vi "DMM Read Dual Display.vi"() -> ()   [LabVIEW 2018]
uses:
  <instrlib>/DMM4/DMM4.lvlib
panel:
  in  "measure":bool
  in  "Reset":bool=TRUE
  out "Measure 2nd Value":string
  in  "Manual Range":dbl=0.5 format="%#.9e"
  in  "Auto Range":bool
  in  "2nd Function":u8(ring)=2 items=["DC Voltage", "AC Voltage", "DC Current", "AC Current", "2-Wire Resistance", "Frequency", "Period", "None"]
  in  "1st Function":u8(ring) items=["DC Voltage", "AC Voltage", "DC+AC Voltage", "DC Current", "AC Current", "DC+AC Current", "2-Wire Resistance", "Frequency", "Period", "Continuity", "Diode", "Temperature", "Capacitance"]
  out "error out":errorcluster
  out "Measure 1st Value":string
  in  "Stop":bool
  out "Boolean":bool
  in  "Detector Rate":u16(ring)=2 items=["SLOW", "MID", "FAST"]
  in  "Manual Range":dbl=1000.0 format="%#.9e"
  in  "Auto Range":bool
  out "ID Return String":string
  in  "Configure RS232 Baud Rate":u32(ring)=115200 items=["9600"=9600, "19200"=19200, "38400"=38400, "57600"=57600, "115200"=115200]
  in  "VISA resource name":refnum<visa-resource-name>="COM15"
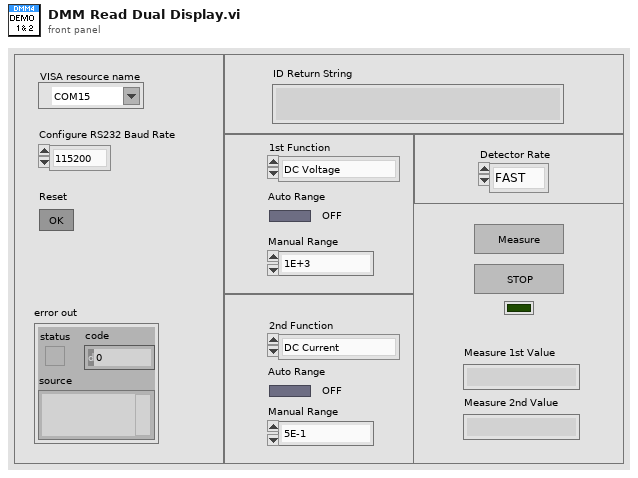
[diagram p1: front panel]
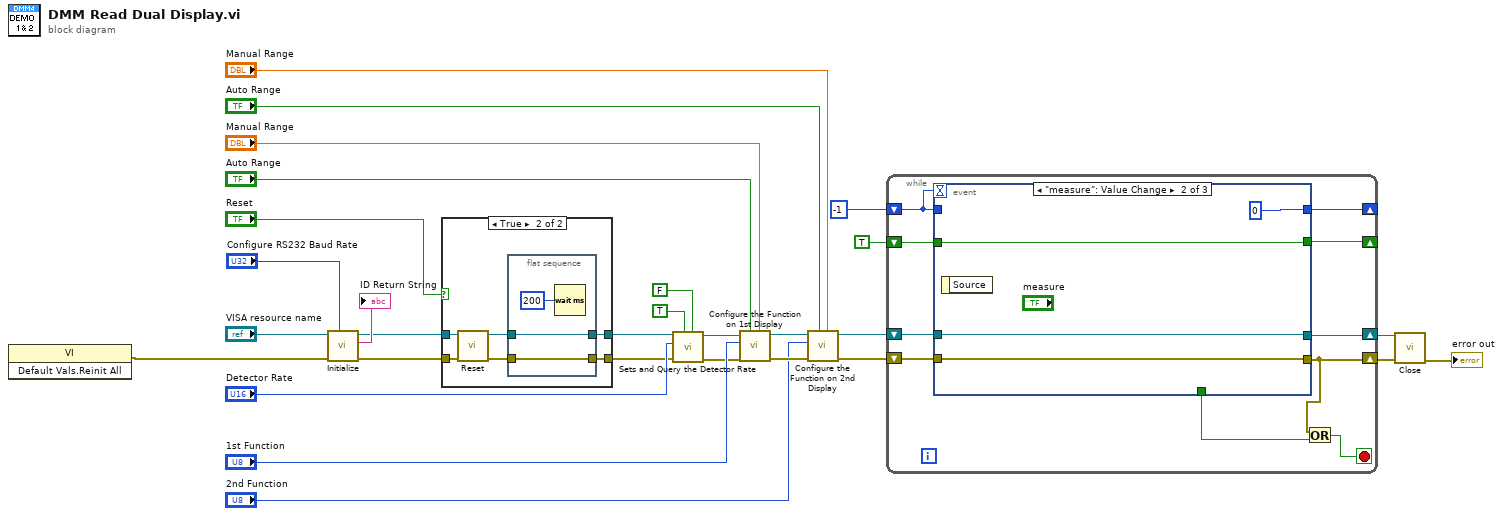
[diagram p0: block diagram]
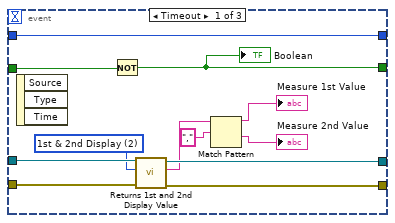
[diagram p3: hidden frame]
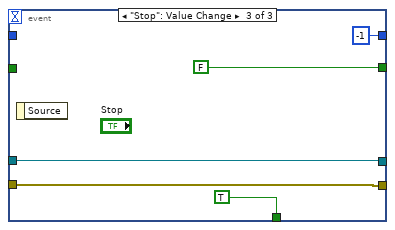
[diagram p4: hidden frame]
diagram:
  n1 = invoke class="VI" method="Default Vals.Reinit All"() -> (error out=w1:errorcluster)  [unwired: 3 in, 2 out]
  n2 = call <instrlib>:"Initialize.vi"("Configure RS232 Baud Rate"="Configure RS232 Baud Rate", "error in (no error)"=w1, "VISA resource name"="VISA resource name") -> ("error out"=w20:errorcluster, "ID Return String"=→"ID Return String":string, "VISA resource name out"=w21:refnum<visa-resource-name>)  [unwired: 5 in, 1 out]
  n3 = case shown="True" "Reset" {
    tunnel: w21 -> [w31 w37]
    tunnel: w20 -> [w30 w36]
    tunnel: [w31 w34] -> w4
    tunnel: [w30 w32] -> w3
    frame False {
    }
    frame True {
      n4 = call <instrlib>:"Reset.vi"("error in (no error)"=w36, "VISA resource name"=w37) -> ("error out"=w33:errorcluster, "VISA resource name out"=w35:refnum<visa-resource-name>)  [unwired: 8 in]
      n5 = flat-sequence {
        tunnel: w35 -> [w39]
        tunnel: [w39] -> w34
        tunnel: w33 -> [w38]
        tunnel: [w38] -> w32
        frame #0 {
          n6 = Wait (ms)(milliseconds to wait=u32 200) -> ()  [unwired: 1 out]
        }
      }
    }
  }
  n7 = call <instrlib>:"Sets and Query the Detector Rate.vi"("Enable to Query"=FALSE, "Enable to Sets"=TRUE, "error in"=w3, "Detector Rate"="Detector Rate", "VISA resource name"=w4) -> ("error out"=w9:errorcluster, "VISA resource name out"=w10:refnum<visa-resource-name>)  [unwired: 4 in, 1 out]
  n8 = call <instrlib>:"Configure the Function on 1st Display .vi"("Manual Range"="Manual Range", "Enable Auto Range"="Auto Range", "error in"=w9, "Function"="1st Function", "VISA resource name"=w10) -> ("error out"=w17:errorcluster, "VISA resource name out"=w18:refnum<visa-resource-name>)  [unwired: 5 in]
  n9 = call <instrlib>:"Configure the Function on 2nd Display.vi"("Manual Range"="Manual Range", "Enable Auto Range"="Auto Range", "error in"=w17, "Function"="2nd Function", "VISA resource name"=w18) -> ("error out"=w11:errorcluster, "VISA resource name out"=w12:refnum<visa-resource-name>)  [unwired: 5 in]
  n10 = while {
    shift-right: [w46] -> _
    shift-left: TRUE -> [w47]
    shift-right: [w44] -> _
    shift-left: -1 -> [w45]
    shift-right: [w48] -> w24
    shift-left: w12 -> [w50]
    shift-right: [w43] -> w23
    shift-left: w11 -> [w49]
    stop <- w41 stop-if-true
    n11 = event shown="[1] \"measure\": Value Change" {
      selector: _ -> [_ _ _]
      dyn-events: _ -> [_ _ _]
      timeout: w45 -> [_ _ _]
      tunnel: w50 -> [w62 w66 w71]
      tunnel: w49 -> [w61 w65 w69]
      tunnel: [w59 w66 w71] -> w48
      tunnel: [w58 w65 w69] -> w43
      tunnel: w47 -> [w57 w64 _]
      tunnel: [w56 w64 FALSE] -> w46
      tunnel: [_ _ TRUE] -> w42
      tunnel: w45 -> [w51 _ _]
      tunnel: [w51 0 -1] -> w44
      event Timeout {
        w60 = u16 2 items=["1st Display", "2nd Display", "1st & 2nd Display"] ("Sets to Display")
        n12 = event-data() -> ()  [unwired: 1 in, 3 out]
        n13 = Not(x=w57) -> (.not. x?=w56:bool)
        "Boolean" <- w56
        n14 = call <instrlib>:"Returns 1st and 2nd Display Value.vi"("error in"=w61, "Sets to Display"=w60, "VISA resource name"=w62) -> ("error out"=w58:errorcluster, "Return the Value"=w55:string, "VISA resource name out"=w59:refnum<visa-resource-name>)  [unwired: 6 in]
        n15 = Match Pattern(string=w55, regular expression=",") -> (before substring=→"Measure 1st Value":string, after substring=→"Measure 2nd Value":string)  [unwired: 1 in, 2 out]
      }
      event "measure": Value Change {
        n16 = event-data() -> ()  [unwired: 1 in, 1 out]
      }
      event "Stop": Value Change {
        n17 = event-data() -> ()  [unwired: 1 in, 1 out]
      }
    }
    n18 = Or(x=w43, y=w42) -> (x .or. y?=w41:bool)
  }
  n19 = call <instrlib>:"Close.vi"("error in (no error)"=w23, "VISA resource name"=w24) -> ("error out"=→"error out":errorcluster)  [unwired: 9 in]
